vi "SLL DE AO Engine.vi"(8 "error in (no error)":errorcluster) -> (0 "error out":errorcluster)   [LabVIEW 2013]
doc: "Copyright © 2005, Soliton Technologies.\nAll rights reserved."
uses:
  Controls/SLL DE DAQ Engine Options.ctl
  Controls/SLL DE AO Min Max Range Checking Options.ctl
  Controls/SLL DE DAQ Global Options.ctl
  Controls/SLL DE DAQ Global Elements.ctl
  Controls/SLL DE AO Command LV2Global Options.ctl
  Controls/SLL DE AO Global Options.ctl
  Controls/SLL DE AO Response LV2Global Options.ctl
  Controls/SLL DE AO Safe Value Global Options.ctl
  <vilib>/DAQmx/write.llb/DAQmx Write (Analog DBL 1Chan 1Samp).vi
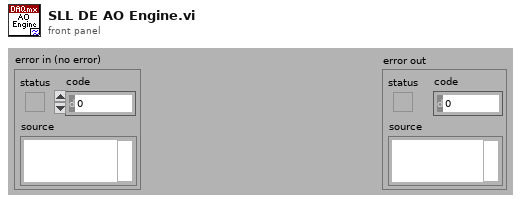
[diagram p1: front panel]
types:
  T1 = typedef "SLL DE DAQ Engine Options.ctl" = enum16{">Init", ">Safe Mode", ">Poll", ">Error", ">Exit", ">Restart", ">DI", ">DO", ">AI", ">AO", ">Start Task", ">Stop Task"}
  T2 = typedef "SLL DE AO Response LV2Global Options.ctl" = enum16{"Initialize", "Send Response", "Check Response", "Close"}
  T3 = typedef "SLL DE AO Global Options.ctl" = enum16{"Init", "Write Line", "Write Array", "Read Line", "Read Array", "Read Full Status", "Restart AO", "Send to Safe Mode", "Stop AO"}
  T4 = typedef "SLL DE AO Command LV2Global Options.ctl" = enum16{"Init/Register Events", "Get Event Refnum", "Fire Event", "Distroy Event"}
  T5 = typedef "SLL DE DAQ Global Elements.ctl" = enum16{"AI Error", "AO Error", "DI Error", "DO Error", "AI Restart", "DI Restart", "AI Running", "AO Running", "DI Running", "DO Running", "DAQ Exit?"}
  T6 = typedef "SLL DE DAQ Global Options.ctl" = enum16{"Init", "Write 1", "Read 1", "Write Array", "Read Array", "Clear"}
  T7 = typedef "SLL DE AO Min Max Range Checking Options.ctl" = enum16{"Initalize Channel Range", "Check Single AO Channel", "Check Multiple AO Channels"}
  T8 = typedef "SLL DE AO Safe Value Global Options.ctl" = enum16{"Read", "Write"}
  T9 = cluster{"Previous AO Data":dbl[], "AO Channels":refnum<k21>[], "Execute For":string}
  T10 = typedef "SLL DE List of Analog Outputs.ctl" = enum16{"None"}
  T11 = enum16{"Left Button", "Center Button", "Right Button", "Window Close"}
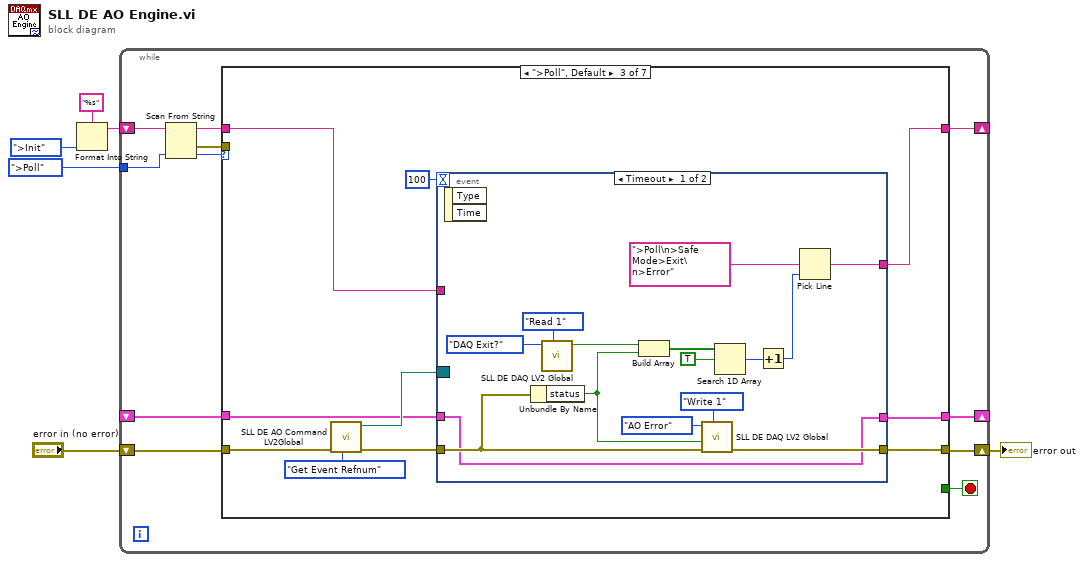
[diagram p0: block diagram]
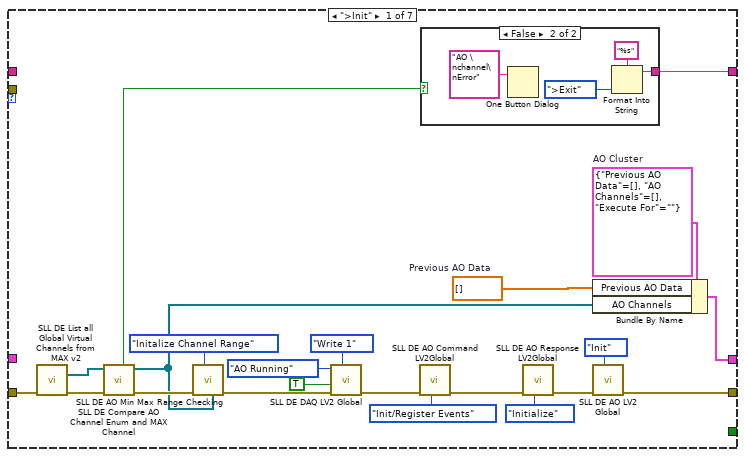
[diagram p2: hidden frame]
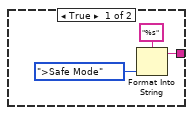
[diagram p3: hidden frame]
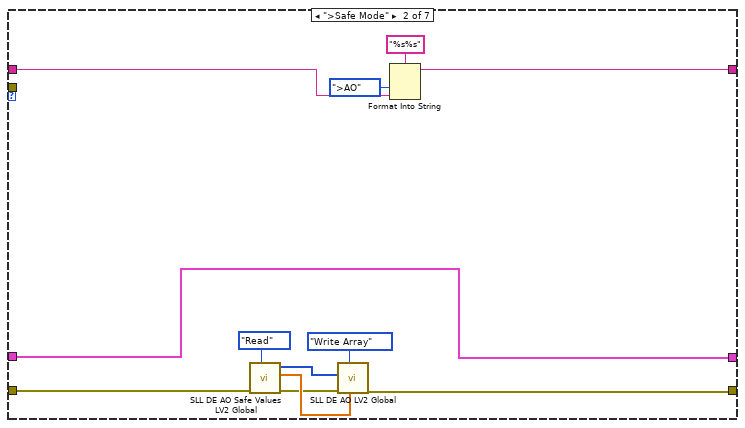
[diagram p4: hidden frame]
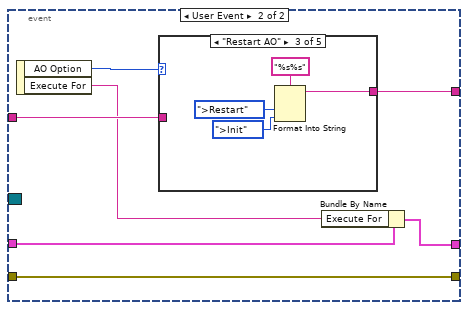
[diagram p5: hidden frame]
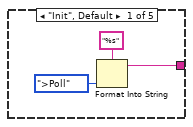
[diagram p6: hidden frame]
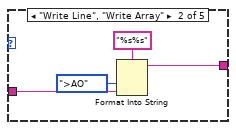
[diagram p7: hidden frame]
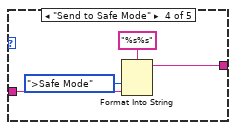
[diagram p8: hidden frame]
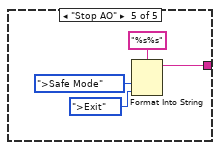
[diagram p9: hidden frame]
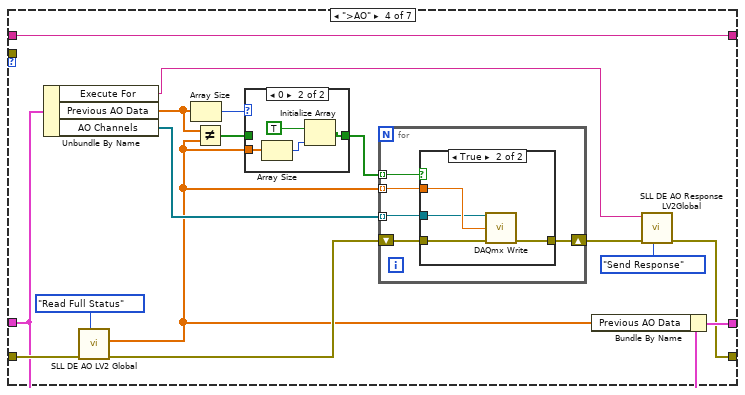
[diagram p10: hidden frame]
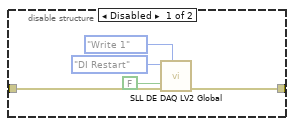
[diagram p14: hidden frame]
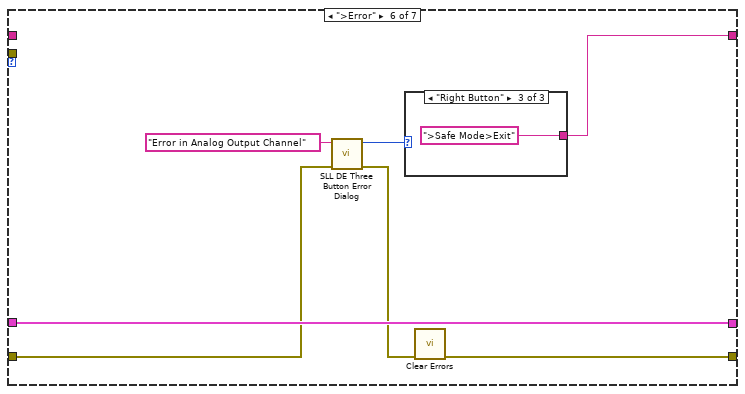
[diagram p15: hidden frame]
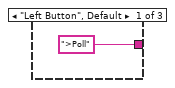
[diagram p16: hidden frame]
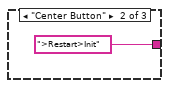
[diagram p17: hidden frame]
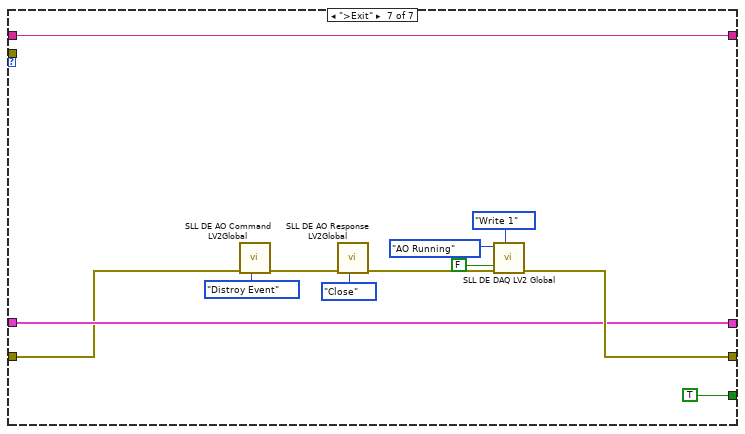
[diagram p18: hidden frame]
diagram:
  n1 = Format Into String(format string="%s", SLL_DE_DAQ_Engine_Options.">Init" ("DAQ Options")) -> (resulting string=w2:string)  [unwired: 2 in, 1 out]
  n2 = while {
    shift-right: [w16] -> w5
    shift-left: "error in (no error)" -> [w17]
    shift-right: [w15] -> _
    shift-left: _ -> [w14]
    shift-right: [w10] -> _
    shift-left: w2 -> [w13]
    tunnel: SLL_DE_DAQ_Engine_Options.">Poll" ("DAQ Options") -> [w7]
    stop <- w9 stop-if-true
    n3 = Scan From String(input string=w13, default 1=w7) -> (remaining string=w12:string, error out=w11:errorcluster, output 1=w8:T1)  [unwired: 3 in, 1 out]
    n4 = case shown="\">Poll\", Default" w8 {
      tunnel: w17 -> [w18 w54 w68 w124 w142 w155 w165]
      tunnel: [w38 w47 w67 w112 w141 w154 w167] -> w16
      tunnel: [w37 w52 w59 w122 w143 w157 w166] -> w15
      tunnel: w14 -> [_ w52 w60 w123 w143 w157 w166]
      tunnel: w12 -> [_ w51 w65 w125 w144 _ w172]
      tunnel: w11 -> [_ _ _ _ _ _ _]
      tunnel: [w39 w50 w66 w125 w144 w152 w172] -> w10
      tunnel: [_ _ _ _ _ _ TRUE] -> w9
      frame ">Init" {
        w29 = T9 {"Previous AO Data"=[], "AO Channels"=[], "Execute For"=""}  # AO Cluster
        w22 = dbl[] []  # Previous AO Data
        n5 = call "SLL DE List all Global Virtual Channels from MAX v2.vi"("error in (no error)"=w18) -> ("error out"=w36:errorcluster, "Analog Output"=w28:refnum<k21>[])  [unwired: 4 in, 5 out]
        n6 = call "SLL DE Compare AO Channel Enum and MAX Channel.vi"("error in (no error)"=w36, "Analog Output Channels"=w28) -> ("error out"=w33:errorcluster, "Channels Out"=w27:refnum<k21>[], "Pass?"=w35:bool)  [unwired: 7 in]
        n7 = call "SLL DE AO Min Max Range Checking.vi"("Analog Output Channels"=w27, "Option"=SLL_DE_AO_Min_Max_Range_Checking_Options."Initalize Channel Range", "error in (no error)"=w33) -> ("error out"=w26:errorcluster)  [unwired: 6 in, 2 out]
        n8 = call "SLL DE DAQ LV2 Global.vi"("Option"=SLL_DE_DAQ_Global_Options."Write 1", "error in (no error)"=w26, "Status In"=TRUE, "Element"=SLL_DE_DAQ_Global_Elements."AO Running") -> ("error out"=w25:errorcluster)  [unwired: 5 in, 2 out]
        n9 = call "SLL DE AO Command LV2Global.vi"("Option"=SLL_DE_AO_Command_LV2Global_Options."Init/Register Events", "Error in (no error)"=w25) -> ("Error out"=w21:errorcluster)  [unwired: 8 in, 1 out]
        n10 = case shown="False" w35 {
          tunnel: [w40 w43] -> w39
          frame True {
            n11 = Format Into String(format string="%s", SLL_DE_DAQ_Engine_Options.">Safe Mode" ("DAQ Options")) -> (resulting string=w40:string)  [unwired: 2 in, 1 out]
          }
          frame False {
            n12 = One Button Dialog(message="AO \nchannel\nError") -> ()  [unwired: 1 in, 1 out]
            n13 = Format Into String(format string="%s", SLL_DE_DAQ_Engine_Options.">Exit" ("DAQ Options")) -> (resulting string=w43:string)  [unwired: 2 in, 1 out]
          }
        }
        n14 = call "SLL DE AO Response LV2Global.vi"("Option"=SLL_DE_AO_Response_LV2Global_Options."Initialize", "Error in (no error)"=w21) -> ("Error out"=w20:errorcluster)  [unwired: 8 in, 1 out]
        n15 = Bundle By Name(cluster=w29, "Previous AO Data"=w22, "AO Channels"=w27) -> (w37:T9)
        n16 = call "SLL DE AO LV2 Global.vi"("AO Option"=SLL_DE_AO_Global_Options."Init", "error in (no error)"=w20) -> ("error out"=w38:errorcluster)  [unwired: 6 in, 3 out]
      }
      frame ">Safe Mode" {
        n17 = call "SLL DE AO Safe Values LV2 Global.vi"("Cases"=SLL_DE_AO_Safe_Value_Global_Options."Read", "error in (no error)"=w54) -> ("error out"=w55:errorcluster, "Value Array Out"=w56:dbl[], "Elements Out"=w57:T10[])  [unwired: 7 in]
        n18 = call "SLL DE AO LV2 Global.vi"("AO value Array"=w56, "AO Option"=SLL_DE_AO_Global_Options."Write Array", "error in (no error)"=w55, "AO Channel Name Array"=w57) -> ("error out"=w47:errorcluster)  [unwired: 4 in, 3 out]
        n19 = Format Into String(format string="%s%s", SLL_DE_DAQ_Engine_Options.">AO" ("DAQ Options"), w51) -> (resulting string=w50:string)  [unwired: 2 in, 1 out]
      }
      frame ">Poll", Default {
        n20 = call "SLL DE AO Command LV2Global.vi"("Option"=SLL_DE_AO_Command_LV2Global_Options."Get Event Refnum", "Error in (no error)"=w68) -> ("Error out"=w64:errorcluster, "Event Registration Refnum"=w63:refnum<event-registration>)  [unwired: 8 in]
        n21 = event shown="[0] Timeout" {
          selector: w63 -> [_ _]
          dyn-events: _ -> [_ _]
          timeout: 100 -> [_ _]
          tunnel: w64 -> [w74 w89]
          tunnel: [w75 w89] -> w67
          tunnel: [w73 w87] -> w66
          tunnel: w65 -> [_ w88]
          tunnel: w60 -> [w72 w86]
          tunnel: [w72 w84] -> w59
          event Timeout {
            n22 = event-data() -> ()  [unwired: 1 in, 2 out]
            n23 = Unbundle By Name(w74) -> ("status"=w83:bool)
            n24 = call "SLL DE DAQ LV2 Global.vi"("Option"=SLL_DE_DAQ_Global_Options."Read 1", "Element"=SLL_DE_DAQ_Global_Elements."DAQ Exit?") -> ("Status Out"=w69:bool)  [unwired: 7 in, 2 out]
            n25 = Build Array(w69, w83) -> (w77:bool[])
            n26 = call "SLL DE DAQ LV2 Global.vi"("Option"=SLL_DE_DAQ_Global_Options."Write 1", "error in (no error)"=w74, "Status In"=w83, "Element"=SLL_DE_DAQ_Global_Elements."AO Error") -> ("error out"=w75:errorcluster)  [unwired: 5 in, 2 out]
            n27 = Search 1D Array(1D array=w77, element=TRUE) -> (index of element=w79:i32)  [unwired: 1 in]
            n28 = Increment(x=w79) -> (x+1=w80:i32)
            n29 = Pick Line(multi-line string=">Poll\n>Safe Mode>Exit\n>Error", line index=w80) -> (output string=w73:string)  [unwired: 1 in]
          }
          event User Event {
            n30 = event-data() -> ("AO Option"=w90:T3, "Execute For"=w85:string)  [unwired: 1 in]
            n31 = case shown="\"Restart AO\"" w90 {
              tunnel: w88 -> [_ w95 _ w103 _]
              tunnel: [w91 w94 w98 w102 w107] -> w87
              frame "Init", Default {
                n32 = Format Into String(format string="%s", SLL_DE_DAQ_Engine_Options.">Poll" ("DAQ Options")) -> (resulting string=w91:string)  [unwired: 2 in, 1 out]
              }
              frame "Write Line", "Write Array" {
                n33 = Format Into String(format string="%s%s", SLL_DE_DAQ_Engine_Options.">AO" ("DAQ Options"), w95) -> (resulting string=w94:string)  [unwired: 2 in, 1 out]
              }
              frame "Restart AO" {
                n34 = Format Into String(format string="%s%s", SLL_DE_DAQ_Engine_Options.">Restart" ("DAQ Options"), SLL_DE_DAQ_Engine_Options.">Init" ("DAQ Options")) -> (resulting string=w98:string)  [unwired: 2 in, 1 out]
              }
              frame "Send to Safe Mode" {
                n35 = Format Into String(format string="%s%s", SLL_DE_DAQ_Engine_Options.">Safe Mode" ("DAQ Options"), w103) -> (resulting string=w102:string)  [unwired: 2 in, 1 out]
              }
              frame "Stop AO" {
                n36 = Format Into String(format string="%s%s", SLL_DE_DAQ_Engine_Options.">Safe Mode" ("DAQ Options"), SLL_DE_DAQ_Engine_Options.">Exit" ("DAQ Options")) -> (resulting string=w107:string)  [unwired: 2 in, 1 out]
              }
            }
            n37 = Bundle By Name(cluster=w86, "Execute For"=w85) -> (w84:T9)
          }
        }
      }
      frame ">AO" {
        n38 = Unbundle By Name(w123) -> ("Execute For"=w111:string, "Previous AO Data"=w118:dbl[], "AO Channels"=w120:refnum<k21>[])
        n39 = call "SLL DE AO LV2 Global.vi"("AO Option"=SLL_DE_AO_Global_Options."Read Full Status", "error in (no error)"=w124) -> ("error out"=w119:errorcluster, "Analog Output Array Value"=w114:dbl[])  [unwired: 6 in, 2 out]
        n40 = Array Size(array=w118) -> (size(s)=w117:i32)
        n41 = Not Equal?(x=w118, y=w114) -> (x != y?=w116:bool[])
        n42 = case shown="0" w117 {
          tunnel: w116 -> [w126 _]
          tunnel: [w126 w129] -> w115
          tunnel: w114 -> [_ w128]
          frame Default {
          }
          frame 0 {
            n43 = Array Size(array=w128) -> (size(s)=w127:i32)
            n44 = Initialize Array(TRUE, w127) -> (w129:bool[])
          }
        }
        n45 = for {
          tunnel: w115 -> [w132] mode=indexing
          tunnel: w114 -> [w135] mode=indexing
          shift-right: [w133] -> w113
          shift-left: w119 -> [w134]
          tunnel: w120 -> [w131] mode=indexing
          n46 = case shown="True" w132 {
            tunnel: w135 -> [_ w138]
            tunnel: w134 -> [w136 w140]
            tunnel: [w136 w139] -> w133
            tunnel: w131 -> [_ w137]
            frame False {
            }
            frame True {
              n47 = call-poly <vilib>:"DAQmx Write.vi"("task/channels in"=w137, "data"=w138, "error in"=w140) -> ("error out"=w139:errorcluster)  [unwired: 10 in, 2 out]
            }
          }
        }
        n48 = Bundle By Name(cluster=w123, "Previous AO Data"=w114) -> (w122:T9)
        n49 = call "SLL DE AO Response LV2Global.vi"("Option"=SLL_DE_AO_Response_LV2Global_Options."Send Response", "Error in (no error)"=w113, "Executed For?"=w111) -> ("Error out"=w112:errorcluster)  [unwired: 7 in, 1 out]
      }
      frame ">Restart" {
        n50 = disable-structure shown="Enabled" {
          disable-tunnel: w142 -> [w146 w150]
          disable-tunnel: [w145 w150] -> w141
          frame Disabled {
            n51 = call "SLL DE DAQ LV2 Global.vi"("Option"=SLL_DE_DAQ_Global_Options."Write 1", "error in (no error)"=w146, "Status In"=FALSE, "Element"=SLL_DE_DAQ_Global_Elements."DI Restart") -> ("error out"=w145:errorcluster)  [unwired: 5 in, 2 out]
          }
          frame Enabled {
          }
        }
      }
      frame ">Error" {
        n52 = call "SLL DE Three Button Error Dialog.vi"("Error In"=w155, "Window Title"="Error in Analog Output Channel") -> ("Error Out"=w151:errorcluster, "Which Button?"=w153:T11)  [unwired: 8 in]
        n53 = case shown="\"Right Button\"" w153 {
          tunnel: [">Poll" ("Window Title") ">Restart>Init" ("Window Title") ">Safe Mode>Exit" ("Window Title")] -> w152
          frame "Left Button", Default {
          }
          frame "Center Button" {
          }
          frame "Right Button" {
          }
        }
        n54 = call <vilib>:"Clear Errors.vi"("error in (no error)"=w151) -> ("error out"=w154:errorcluster)  [unwired: 6 in]
      }
      frame ">Exit" {
        n55 = call "SLL DE AO Command LV2Global.vi"("Option"=SLL_DE_AO_Command_LV2Global_Options."Distroy Event", "Error in (no error)"=w165) -> ("Error out"=w162:errorcluster)  [unwired: 8 in, 1 out]
        n56 = call "SLL DE AO Response LV2Global.vi"("Option"=SLL_DE_AO_Response_LV2Global_Options."Close", "Error in (no error)"=w162) -> ("Error out"=w161:errorcluster)  [unwired: 8 in, 1 out]
        n57 = call "SLL DE DAQ LV2 Global.vi"("Option"=SLL_DE_DAQ_Global_Options."Write 1", "error in (no error)"=w161, "Status In"=FALSE, "Element"=SLL_DE_DAQ_Global_Elements."AO Running") -> ("error out"=w167:errorcluster)  [unwired: 5 in, 2 out]
      }
    }
  }
  "error out" <- w5
